vi "CD Init_Prepare Inline Data_Compute Index from CWD1 NOT for Broadcast.vi"(11 "message":T1 {"Timestamp Channel Data Reference" format="%.0x"; "Status Channel Data Refs" format="%.0x"; "param item refs" format="%.0x"; "param Block Data Refs"."Data Reference" format="%.0x"}) -> (0 "RT to RT?":bool, 1 "Index 1":u32, 2 "Broadcast?":bool, 3 "Index 0":u16, 4 "Index 2":u16, 5 "CWD1.SA":i8)   [LabVIEW 2020, in "Ballard MIL-1553 Engine.lvlib"]
uses:
  Ballard MIL-1553 Engine.lvlib
  Shared/Controls and Global/RT Message.ctl
  Shared/Controls and Global/RT messageType.ctl
  Shared/Controls and Global/RT CWD1.ctl
  Shared/Controls and Global/RT CWD2.ctl
  <vilib>/NI VeriStand/Custom Device API/Data Reference.ctl
  <vilib>/NI VeriStand/Custom Device API/Custom Device Item Ref.ctl
  <vilib>/NI VeriStand/Custom Device API/Block Data Reference.ctl
  System Explorer/SubVIs/Parse Parameters File/param_map_sysdef_type.ctl
  Azdo/emea-ni-vscd_Configurator/source/ConfiguratorConsumer/Helpers/Configuration/_typedefs/param_type.ctl
  Azdo/emea-ni-vscd_Configurator/source/ConfiguratorConsumer/Helpers/Configuration/_typedefs/param_signalType_type.ctl
  Azdo/emea-ni-vscd_Configurator/source/ConfiguratorConsumer/Helpers/Configuration/_typedefs/param_encoding_type.ctl
  <vilib>/NI VeriStand/Custom Device API/Custom Device API.lvlib
  Shared/Ballard 1553 Shared.lvlib
  Azdo/emea-ni-vscd_Configurator/source/ConfiguratorConsumer/Helpers/Configuration/Configuration_Helper.lvlib
  System Explorer/Ballard 1553 System Explorer.lvlib
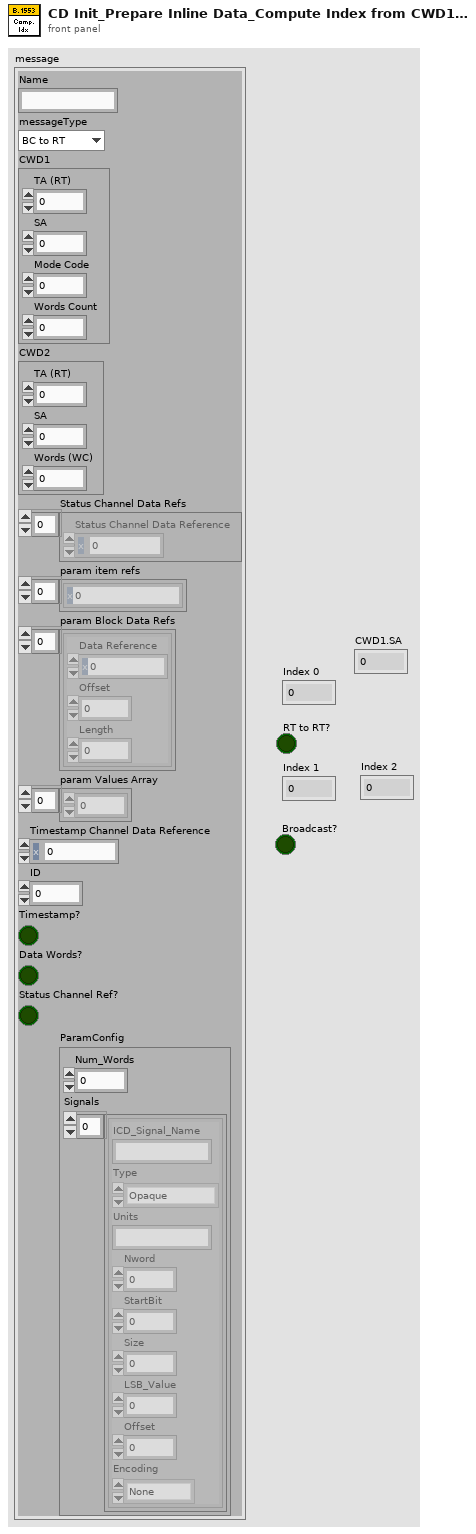
[diagram p1: front panel]
types:
  T1 = typedef "Ballard 1553 Shared.lvlib/RT Message.ctl" = cluster{"Name":string, "messageType":T2, "CWD1":T3, "CWD2":T4, "Status Channel Data Refs":T5[], "param item refs":T6[], "param Block Data Refs":T7[], "param Values Array":u16[], "Timestamp Channel Data Reference":T5, "ID":i32, "Timestamp?":bool, "Data Words?":bool, "Status Channel Ref?":bool, "ParamConfig":T8}
  T2 = typedef "Ballard 1553 Shared.lvlib/RT messageType.ctl" = enum16{"BC to RT", "RT to BC", "RT to RT", "MC (Rx)", "MC (Tx)"}
  T3 = typedef "Ballard 1553 Shared.lvlib/RT CWD1.ctl" = cluster{"TA (RT)":i8, "SA":i8, "Mode Code":i8, "Words Count":i8}
  T4 = typedef "Ballard 1553 Shared.lvlib/RT CWD2.ctl" = cluster{"TA (RT)":i8, "SA":i8, "Words (WC)":i8}
  T5 = typedef "Custom Device API.lvlib/Data Reference.ctl" = i32
  T6 = typedef "Custom Device API.lvlib/Custom Device Item Ref.ctl" = u64
  T7 = typedef "Custom Device API.lvlib/Block Data Reference.ctl" = cluster{"Data Reference":T5, "Offset":u64, "Length":u64}
  T8 = typedef "Ballard 1553 System Explorer.lvlib/param_map_sysdef_type.ctl" = cluster{"Num_Words":u8, "Signals":T9[]}
  T9 = typedef "Configuration_Helper.lvlib/param_type.ctl" = cluster{"ICD_Signal_Name":string, "Type":T10, "Units":string, "Nword":i32, "StartBit":i32, "Size":i32, "LSB_Value":dbl, "Offset":i32, "Encoding":T11}
  T10 = typedef "Configuration_Helper.lvlib/param_signalType_type.ctl" = enum16{"Opaque", "Enum", "Float", "Integer", "Bcd", "Bool"}
  T11 = typedef "Configuration_Helper.lvlib/param_encoding_type.ctl" = enum16{"None", "2-complement", "Unsigned"}
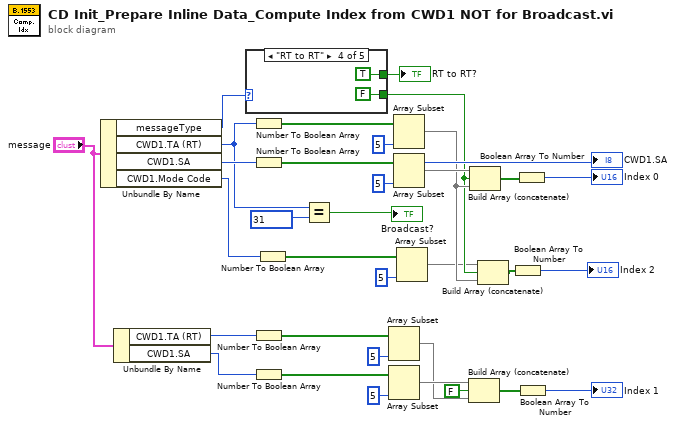
[diagram p0: block diagram]
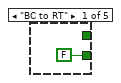
[diagram p2: hidden frame]
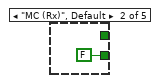
[diagram p3: hidden frame]
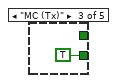
[diagram p4: hidden frame]
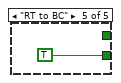
[diagram p5: hidden frame]
diagram:
  n1 = Unbundle By Name("message") -> ("messageType"=w26:T2, "CWD1.TA (RT)"=w11:i8, "CWD1.SA"=w27:i8, "CWD1.Mode Code"=w6:i8)
  "CWD1.SA" <- w27
  n2 = Unbundle By Name("message") -> ("CWD1.TA (RT)"=w19:i8, "CWD1.SA"=w18:i8)
  n3 = case shown="\"RT to RT\"" w26 {
    tunnel: [FALSE FALSE TRUE FALSE TRUE] -> w7
    tunnel: [_ _ _ TRUE _] -> w25
    frame "BC to RT" {
    }
    frame "MC (Rx)", Default {
    }
    frame "MC (Tx)" {
    }
    frame "RT to RT" {
    }
    frame "RT to BC" {
    }
  }
  "RT to RT?" <- w25
  n4 = Number To Boolean Array(number=w11) -> (Boolean array=w28:bool[])
  n5 = Number To Boolean Array(number=w27) -> (Boolean array=w29:bool[])
  n6 = Number To Boolean Array(number=w19) -> (Boolean array=w23:bool[])
  n7 = Number To Boolean Array(number=w18) -> (Boolean array=w22:bool[])
  n8 = Number To Boolean Array(number=w6) -> (Boolean array=w4:bool[])
  n9 = Equal?(x=w11, y=i8 31) -> (x = y?=→"Broadcast?":bool)
  n10 = Array Subset(array=w23, length=5) -> (w15:bool[])  [unwired: 1 in]
  n11 = Array Subset(array=w22, length=5) -> (w17:bool[])  [unwired: 1 in]
  n12 = Array Subset(array=w28, length=5) -> (w8:bool[])  [unwired: 1 in]
  n13 = Array Subset(array=w29, length=5) -> (w32:bool[])  [unwired: 1 in]
  n14 = Array Subset(array=w4, length=5) -> (w3:bool[])  [unwired: 1 in]
  n15 = Build Array (concatenate)(w17, FALSE, w15) -> (w12:bool[])
  n16 = Build Array (concatenate)(w32, w7, w8) -> (w14:bool[])
  n17 = Build Array (concatenate)(w3, w7, w8) -> (w1:bool[])
  n18 = Boolean Array To Number(Boolean array=w1) -> (number=→"Index 2":u16)
  n19 = Boolean Array To Number(Boolean array=w14) -> (number=→"Index 0":u16)
  n20 = Boolean Array To Number(Boolean array=w12) -> (number=→"Index 1":u32)
